vi "decode access token response.vi"(8 "error in (no error)":errorcluster, 9 "Response":string, 10 "Header":string, 11 "Oauth2.GitHub in":refnum<class "Oauth2.GitHub.lvclass">) -> (0 "error out":errorcluster, 3 "Oauth2.GitHub":refnum<class "Oauth2.GitHub.lvclass">)   [LabVIEW 2020, in "Oauth2.GitHub.lvclass"]
uses:
  Oauth2.GitHub.lvclass
  C:/Data/1_Projects/CIGH_Oauth2/source/Oauth2/Oauth2.lvclass
  Oauth2/Oauth2.lvclass
  OAuthToken/OAuth2 Token Element -- enum.ctl
  OAuthToken/OAuthAccessToken.lvclass
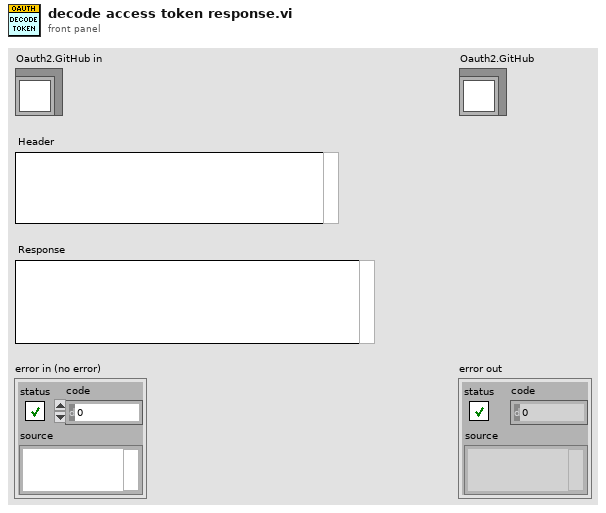
[diagram p1: front panel]
types:
  T1 = typedef "OAuthAccessToken.lvclass/OAuth2 Token Element -- enum.ctl" = enum16{"client_id", "client_secret", "response_type", "scope", "redirect_uri", "error", "error_description", "error_uri", "grant_type", "code", "access_token", "token_type", "expires_in", "username", "password", "refresh_token", "code_challenge", "code_challenge_method", "reverse_proxy_uri", "endpoint element"}
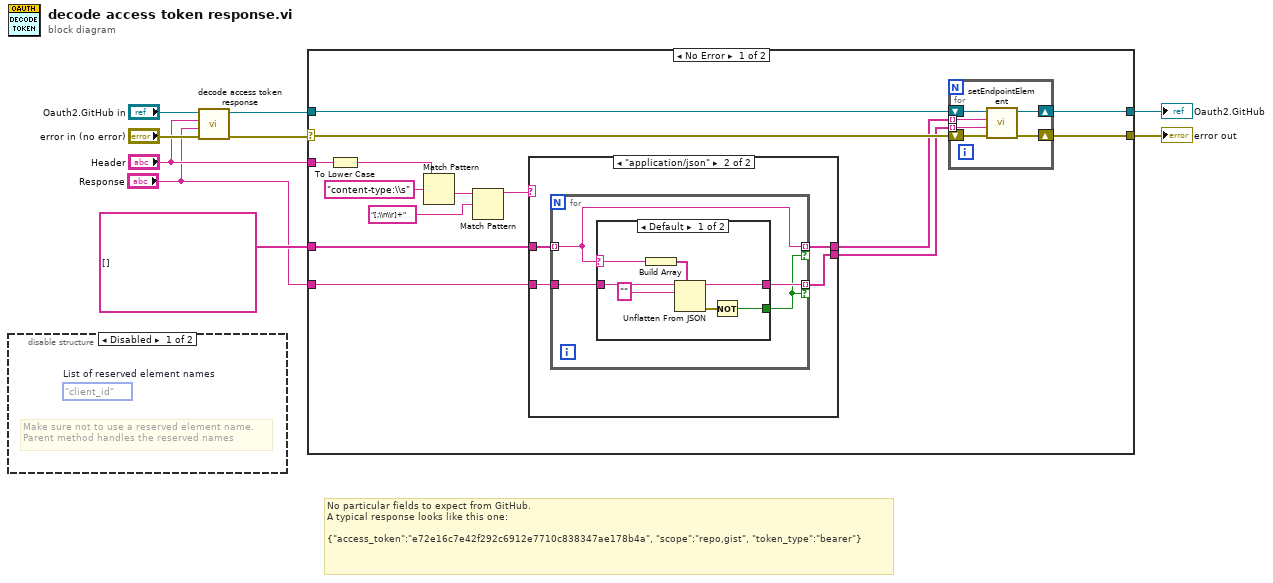
[diagram p0: block diagram]
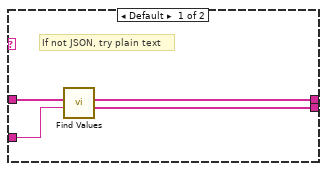
[diagram p3: hidden frame]
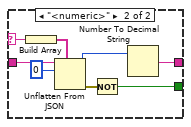
[diagram p4: hidden frame]
diagram:
  # "No particular fields to expect from GitHub.\nA typical response looks like this one:\n\n{\"access_token\":\"e72e16c7e42f292c6912e7710c838347ae178b4a\", \"scope\":\"repo,gist\", \"token_type\":\"bearer\"}"
  n1 = disable-structure shown="Disabled" {
    frame Disabled {
      (unwired) OAuth2_Token_Element_--_enum."client_id"  # List of reserved element names
      # "Make sure not to use a reserved element name.\nParent method handles the reserved names"
    }
    frame Enabled {
    }
  }
  n2 = call-parent "decode access token response.vi"("error in (no error)"="error in (no error)", "Response"="Response", "Header"="Header", "Oauth2 in"="Oauth2.GitHub in") -> ("error out"=w5:errorcluster, "Oauth2"=w6:refnum<class "Oauth2.GitHub.lvclass">)  [unwired: 6 in]
  n3 = case shown="No Error" w5 {
    selector: w5 -> [w19 w58]
    tunnel: [w20 w58] -> w1
    tunnel: [w21 w57] -> w2
    tunnel: w6 -> [w22 w57]
    tunnel: "Response" -> [w23 _]
    tunnel: "Header" -> [w18 _]
    tunnel: string[] [] -> [w13 _]
    frame No Error {
      n4 = To Lower Case(string=w18) -> (all lower case string=w12:string)
      n5 = Match Pattern(string=w12, regular expression="content-type:\\s") -> (after substring=w16:string)  [unwired: 1 in, 3 out]
      n6 = Match Pattern(string=w16, regular expression="[;\\n\\r]+") -> (before substring=w14:string)  [unwired: 1 in, 3 out]
      n7 = case shown="\"application/json\"" w14 {
        tunnel: w23 -> [w33 w37]
        tunnel: w13 -> [w30 w35]
        tunnel: [w32 w34] -> w11
        tunnel: [w31 w36] -> w10
        frame Default {
          # "If not JSON, try plain text"
          n8 = call "Find Values.vi"("Response string"=w33, "keys"=w30) -> ("values"=w31:string[], "keys dup"=w32:string[])  [unwired: 8 in]
        }
        frame "application/json" {
          n9 = for {
            tunnel: w37 -> [w41]
            tunnel: [w40] -> w36 mode=indexing if=w39
            tunnel: w35 -> [w38] mode=indexing
            tunnel: [w38] -> w34 mode=indexing if=w39
            n10 = case shown="Default" w38 {
              selector: w38 -> [w42 w51]
              tunnel: w41 -> [w48 w56]
              tunnel: [w46 w49] -> w40
              tunnel: [w44 w53] -> w39
              frame Default {
                n11 = Build Array(w42) -> (w43:string[])
                n12 = Unflatten From JSON(path=w43, JSON string=w48, type and defaults="") -> (value=w46:string, error out=w45:errorcluster)  [unwired: 4 in]
                n13 = Not(x=w45) -> (.not. x?=w44:bool)
              }
              frame "<numeric>" {
                n14 = Build Array(w51) -> (w52:string[])
                n15 = Unflatten From JSON(path=w52, JSON string=w56, type and defaults=u32 0) -> (value=w50:u32, error out=w54:errorcluster)  [unwired: 4 in]
                n16 = Not(x=w54) -> (.not. x?=w53:bool)
                n17 = Number To Decimal String(number=w50) -> (decimal integer string=w49:string)  [unwired: 1 in]
              }
            }
          }
        }
      }
      n18 = for {
        shift-right: [w28] -> w21
        shift-left: w22 -> [w29]
        shift-right: [w27] -> w20
        shift-left: w19 -> [w26]
        tunnel: w11 -> [w25] mode=indexing
        tunnel: w10 -> [w24] mode=indexing
        n19 = call "setEndpointElement.vi"("error in (no error)"=w26, "Value"=w24, "Endpoint Name"=w25, "Oauth2 in"=w29) -> ("error out"=w27:errorcluster, "Oauth2 out"=w28:refnum<class "Oauth2.GitHub.lvclass">)  [unwired: 6 in]
      }
    }
    frame Error {
    }
  }
  "error out" <- w1
  "Oauth2.GitHub" <- w2
